vi "Calculate Time Constant.vi"(0 "derivative time":sgl, 5 "filter coefficient (NaN)":sgl=nan, 7 "filter coefficient unit (Alpha)":T1 items=["Alpha", "N", "Cutoff Frequency", "Time Constant"]) -> (4 "time constant":sgl)   [LabVIEW 2017]
uses:
  <vilib>/rvi/Analysis/host/Private/PID Filter Coefficient Unit.ctl
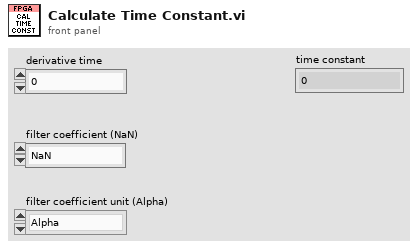
[diagram p1: front panel]
types:
  T1 = typedef "PID Filter Coefficient Unit.ctl" = u8
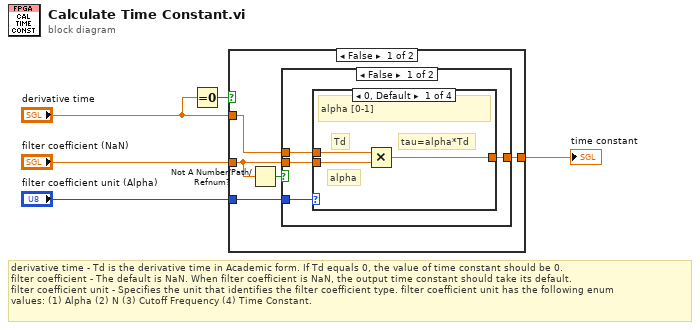
[diagram p0: block diagram]
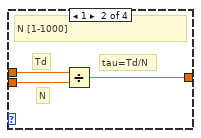
[diagram p2: hidden frame]
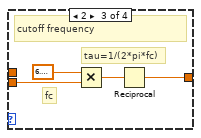
[diagram p3: hidden frame]
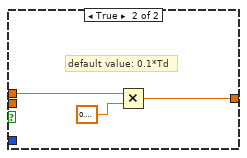
[diagram p5: hidden frame]
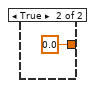
[diagram p6: hidden frame]
diagram:
  # "derivative time - Td is the derivative time in Academic form. If Td equals 0, the value of time constant should be 0.\nfilter coefficient - The default is NaN. When filter coefficient is NaN, the output time constant should take its default.\nfilter coefficient unit - Specifies the unit that identifies the filter coefficient type. filter coefficient unit has the following enum \nvalues: (1) Alpha (2) N (3) Cutoff Frequency (4) Time Constant."
  n1 = Equal To 0?(x="derivative time") -> (x = 0?=w2:bool)
  n2 = case shown="False" w2 {
    tunnel: "filter coefficient unit (Alpha)" -> [w9 _]
    tunnel: "filter coefficient (NaN)" -> [w8 _]
    tunnel: "derivative time" -> [w7 _]
    tunnel: [w6 sgl 0.0 ("filter coefficient (NaN)")] -> w4
    frame False {
      n3 = Not A Number/Path/Refnum?(number/path/refnum=w8) -> (NaN/Path/Refnum?=w10:bool)
      n4 = case shown="False" w10 {
        tunnel: w9 -> [w14 _]
        tunnel: w7 -> [w11 w28]
        tunnel: [w12 w26] -> w6
        tunnel: w8 -> [w13 _]
        frame False {
          n5 = case shown="0, Default" w14 {
            tunnel: w13 -> [w17 w19 w22 w25]
            tunnel: [w16 w20 w21 w25] -> w12
            tunnel: w11 -> [w15 w18 _ _]
            frame 0, Default {
              # "tau=alpha*Td"
              # "Td"
              # "alpha"
              # "alpha [0-1]"
              n6 = Multiply(x=w15, y=w17) -> (x*y=w16:sgl)
            }
            frame 1 {
              # "tau=Td/N"
              # "N"
              # "Td"
              # "N [1-1000]"
              n7 = Divide(x=w18, y=w19) -> (x/y=w20:sgl)
            }
            frame 2 {
              # "tau=1/(2*pi*fc)"
              # "fc"
              # "cutoff frequency"
              n8 = Multiply(x=sgl 6.2831855, y=w22) -> (x*y=w24:sgl)
              n9 = Reciprocal(x=w24) -> (1/x=w21:sgl)
            }
            frame 3 {
              # "tau"
              # "time constant"
            }
          }
        }
        frame True {
          # "default value: 0.1*Td"
          n10 = Multiply(x=w28, y=sgl 0.1) -> (x*y=w26:sgl)
        }
      }
    }
    frame True {
    }
  }
  "time constant" <- w4
